vi "RGB Distance Comparision.vi"(10 "Image 2":path, 11 "Image 1":path) -> (3 "RGB Distance":dbl)   [LabVIEW 2015, in "RGB Distance Comparison.lvclass"]
uses:
  RGB Distance Comparison.lvclass
  Image Comparison/Image Comparison.lvclass
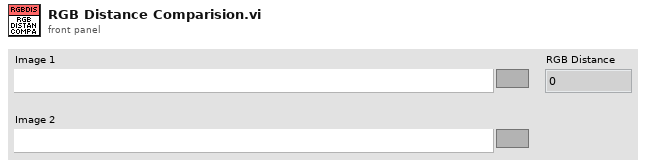
[diagram p1: front panel]
types:
  T1 = typedef "imagedata.ctl" = cluster{"image type":i32, "image depth":i32, "image":u8[], "mask":u8[], "colors":u32[], "Rectangle":cluster{"left":i16, "top":i16, "right":i16, "bottom":i16}}
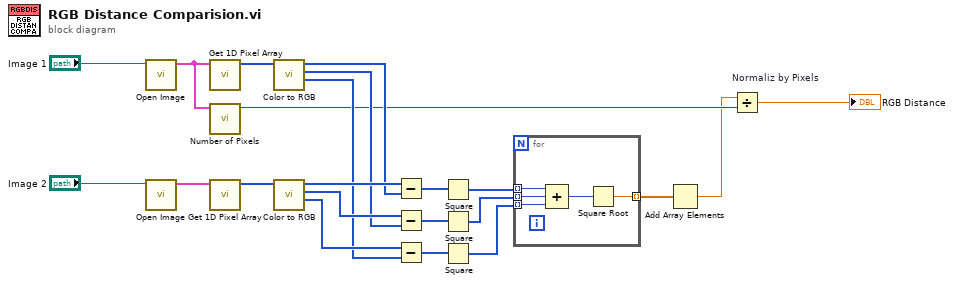
[diagram p0: block diagram]
diagram:
  n1 = call "Open Image.vi"("Image"="Image 1") -> ("image data"=w4:T1)  [unwired: 9 in, 1 out]
  n2 = call "Open Image.vi"("Image"="Image 2") -> ("image data"=w20:T1)  [unwired: 9 in, 1 out]
  n3 = call "Get 1D Pixel Array.vi"("image data"=w4) -> ("1D Pixel Array"=w19:u32[])  [unwired: 10 in]
  n4 = call "Number of Pixels.vi"("image data"=w4) -> ("Number of Pixels"=w3:u64)  [unwired: 10 in]
  n5 = call "Get 1D Pixel Array.vi"("image data"=w20) -> ("1D Pixel Array"=w18:u32[])  [unwired: 10 in]
  n6 = call "Color to RGB.vi"("1D Pixel Array"=w19) -> ("Blue[]"=w12:u8[], "Green[]"=w14:u8[], "Red[]"=w16:u8[])  [unwired: 8 in]
  n7 = call "Color to RGB.vi"("1D Pixel Array"=w18) -> ("Blue[]"=w13:u8[], "Green[]"=w15:u8[], "Red[]"=w17:u8[])  [unwired: 8 in]
  n8 = Subtract(x=w17, y=w16) -> (x-y=w11:u8[])
  n9 = Subtract(x=w15, y=w14) -> (x-y=w10:u8[])
  n10 = Subtract(x=w13, y=w12) -> (x-y=w9:u8[])
  n11 = Square(x=w11) -> (x^2=w8:u8[])
  n12 = Square(x=w10) -> (x^2=w7:u8[])
  n13 = Square(x=w9) -> (x^2=w6:u8[])
  n14 = for {
    tunnel: w8 -> [w27] mode=indexing
    tunnel: w7 -> [w26] mode=indexing
    tunnel: w6 -> [w25] mode=indexing
    tunnel: [w23] -> w5 mode=indexing
    n15 = Compound Arithmetic op=ADD(w27, w26, w25) -> (w24:u8)
    n16 = Square Root(x=w24) -> (sqrt(x)=w23:dbl)
  }
  n17 = Add Array Elements(numeric array=w5) -> (sum=w2:dbl)
  n18 = Divide "Normaliz by Pixels"(x=w2, y=w3) -> (x/y=→"RGB Distance":dbl)
